vi "CCE RRMA P03 SubVI05.vi"(9 "q":dbl, 10 "p":dbl, 11 "Image Data":u8[][](array[numeric])) -> (3 "m normalizado":dbl)   [LabVIEW 2020]
doc: "Ceballos Conde Emanuel Rodríguez Ramírez Miguel Ángel 4MV6 Sistemas de visión artificial 2022/1\neste vi permite obtener el momento normalizado"
panel:
  # "Ceballos Conde Emanuel\nRodríguez Ramírez Miguel Ángel\n4MV6\nSistemas de visión artificial\n2022/1"
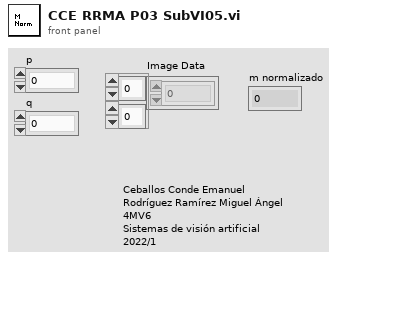
[diagram p1: front panel]
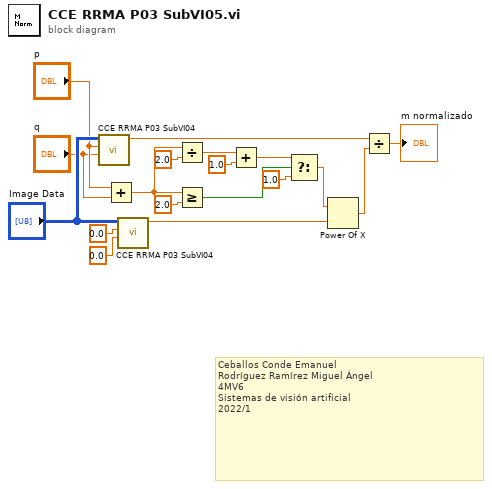
[diagram p0: block diagram]
diagram:
  # "Ceballos Conde Emanuel\nRodríguez Ramírez Miguel Ángel\n4MV6\nSistemas de visión artificial\n2022/1"
  n1 = call "CCE RRMA P03 SubVI04.vi"("q"="q", "p"="p", "Image Data"="Image Data") -> ("MC"=w5:dbl)  [unwired: 8 in]
  n2 = Add(x="p", y="q") -> (x+y=w10:dbl)
  n3 = call "CCE RRMA P03 SubVI04.vi"("q"=0.0, "p"=0.0, "Image Data"="Image Data") -> ("MC"=w4:dbl)  [unwired: 8 in]
  n4 = Divide(x=w10, y=2.0) -> (x/y=w8:dbl)
  n5 = Greater Or Equal?(x=w10, y=2.0) -> (x >= y?=w12:bool)
  n6 = Add(x=w8, y=1.0) -> (x+y=w9:dbl)
  n7 = Select(t=w9, s=w12, f=1.0) -> (s? t:f=w3:dbl)
  n8 = Power Of X(1:w4, 2:w3) -> (0:w2:dbl)
  n9 = Divide(x=w5, y=w2) -> (x/y=→"m normalizado":dbl)
